vi "parseAttributeValue.vi"(8 "error in (no error)":errorcluster, 10 "XMLString in":string, 11 "AttributeReader in":refnum<class "XMLAttributeParser.lvclass">) -> (0 "error out":errorcluster, 2 "ParsedValues":string[](array[string]), 3 "AttributeReader out":refnum<class "XMLAttributeParser.lvclass">)   [LabVIEW 2014, in "XML.lvlib" / "XMLAttributeParser.lvclass"]
doc: "This method finds anything in the open tag of the form (inside the square brackets) [\"AttributeValue\"], throws away the quotation marks and parses the value. It can handle single or double quotes."
uses:
  <userlib>/Common/XML/XMLAttributeParser/XMLAttributeParser.lvclass
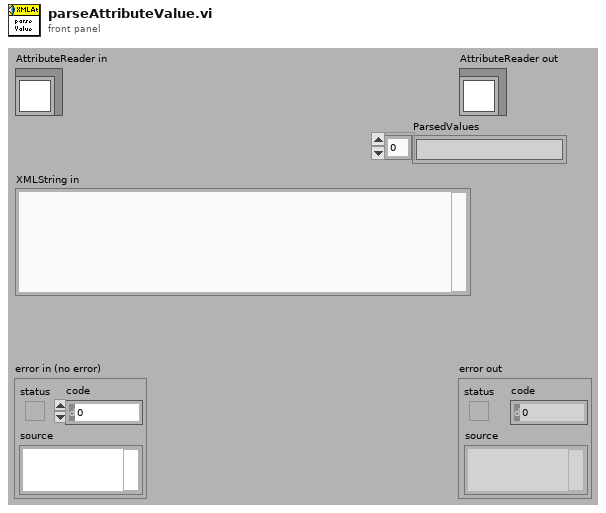
[diagram p1: front panel]
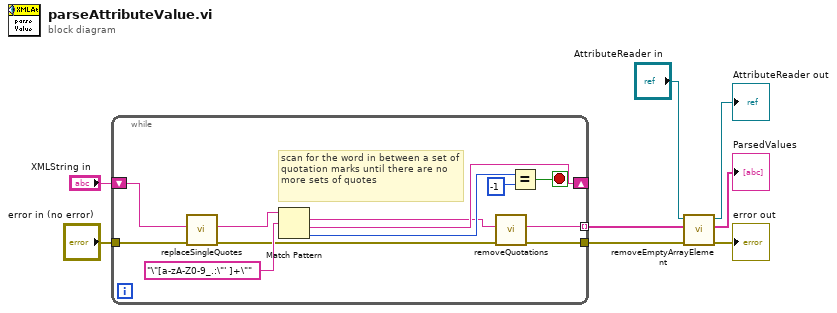
[diagram p0: block diagram]
diagram:
  n1 = while {
    shift-right: [w17] -> _
    shift-left: "XMLString in" -> [w12]
    tunnel: [w15] -> w7 mode=indexing
    tunnel: "error in (no error)" -> [w10]
    tunnel: [w14] -> w6
    stop <- w13 stop-if-true
    # "scan for the word in between a set of quotation marks until there are no more sets of quotes"
    n2 = call <userlib>:"replaceSingleQuotes.vi"("error in (no error)"=w10, "XMLIn"=w12) -> ("error out"=w9:errorcluster, "DoubleQuoteXML"=w11:string)  [unwired: 7 in, 1 out]
    n3 = Match Pattern(string=w11, regular expression="\"[a-zA-Z0-9_.:\"' ]+\"") -> (match substring=w16:string, after substring=w17:string, offset past match=w19:i32)  [unwired: 1 in, 1 out]
    n4 = call <userlib>:"removeQuotations.vi"("error in (no error)"=w9, "quoteIn"=w16) -> ("error out"=w14:errorcluster, "quoteOut"=w15:string)  [unwired: 7 in, 1 out]
    n5 = Equal?(x=w19, y=-1) -> (x = y?=w13:bool)
  }
  n6 = call <userlib>:"removeEmptyArrayElement.vi"("error in (no error)"=w6, "Array in"=w7, "AttributeReader in"="AttributeReader in") -> ("error out"=→"error out":errorcluster, "Array out"=→"ParsedValues":string[], "AttributeReader out"=→"AttributeReader out":refnum<class "XMLAttributeParser.lvclass">)  [unwired: 6 in]
